vi "Write String.vi"(7 "Channel Index":i32, 8 "error in (no error)":errorcluster, 10 "Data":string, 11 "CIFCorePlugin in":refnum<class "CIFCorePlugin.lvclass">) -> (0 "error out":errorcluster, 3 "CIFCorePlugin out":refnum<class "CIFCorePlugin.lvclass">)   [LabVIEW 2021, in "CIFCorePlugin.lvclass"]
uses:
  CIFCorePlugin.lvclass
  CIFCorePlugin.lvclass/CIFCorePlugin.ctl
  <vilib>/CIF Foundation/CIF Channels Core/CIFChannels/CIFChannels.lvclass
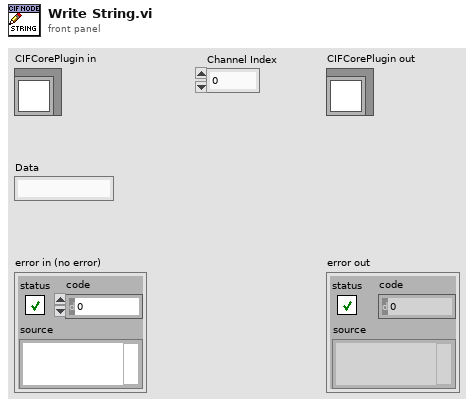
[diagram p1: front panel]
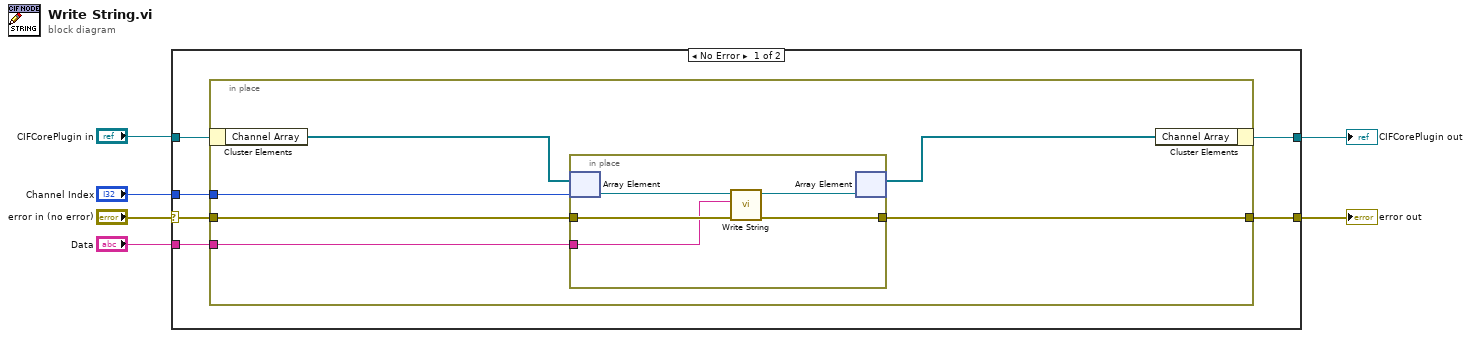
[diagram p0: block diagram]
diagram:
  n1 = case shown="No Error" "error in (no error)" {
    selector: "error in (no error)" -> [w12 w25]
    tunnel: [w11 w25] -> w3
    tunnel: [w8 w24] -> w4
    tunnel: "CIFCorePlugin in" -> [w9 w24]
    tunnel: "Data" -> [w10 _]
    tunnel: "Channel Index" -> [w7 _]
    frame No Error {
      n2 = in-place {
        in-place-border: w12 -> [w16]
        in-place-border: [w15] -> w11
        in-place-border: w10 -> [w18]
        in-place-border: w7 -> [w17]
        n3 = in-place-cluster #1(w9) -> ("Channel Array"=w14:refnum<class "CIFChannels.lvclass">[])
        n4 = in-place {
          in-place-border: w16 -> [w21]
          in-place-border: [w20] -> w15
          in-place-border: w18 -> [w19]
          n5 = in-place-array #2(w14, w17) -> (w23:refnum<class "CIFChannels.lvclass">)
          n6 = call-dynamic "Write String.vi"("error in (no error)"=w21, "Data"=w19, "CIFChannels in"=w23) -> ("error out"=w20:errorcluster, "CIFChannels out"=w22:refnum<class "CIFChannels.lvclass">)  [unwired: 6 in, 1 out]
          n7 = in-place-array #2(w22) -> (w13:refnum<class "CIFChannels.lvclass">[])  [unwired: 1 out]
        }
        n8 = in-place-cluster #1("Channel Array"=w13) -> (w8:refnum<class "CIFCorePlugin.lvclass">)
      }
    }
    frame Error {
    }
  }
  "error out" <- w3
  "CIFCorePlugin out" <- w4
